vi "Thermotron 8800.vi"() -> ()   [LabVIEW 2023, in "Thermotron 8800.lvlib"]
doc: "Example vi that utilizes VISA for communication. Initializes and resets 8800 chamber controller, gets the version information, starts the chamber controller in manual mode and changes the setpoint for channel 1 process variable from zero to 10 in one degree C steps while reading back the process variable and setpoint. Finally, the chamber controller is put into stop mode, errors are handled and the example vi is closed."
uses:
  Thermotron 8800.lvlib
  Private/get set.ctl
  Private/AnalogInputChannelNumber 1-4.ctl
panel:
  in  "stop":bool
  out "Loop Count":i32
  out "PVAR1 value":string
  out "SETP1 value":string
  out "ID result":string
  out "error out":errorcluster
  in  "VISA resource name":refnum<visa-resource-name>="TCPIP::127.0.0.1::8888::SOCKET"
  in  "error in (no error)":errorcluster
  # "TCPIP::192.168.4.118::8888::SOCKET"
  # "GPIB0::1::INSTR"
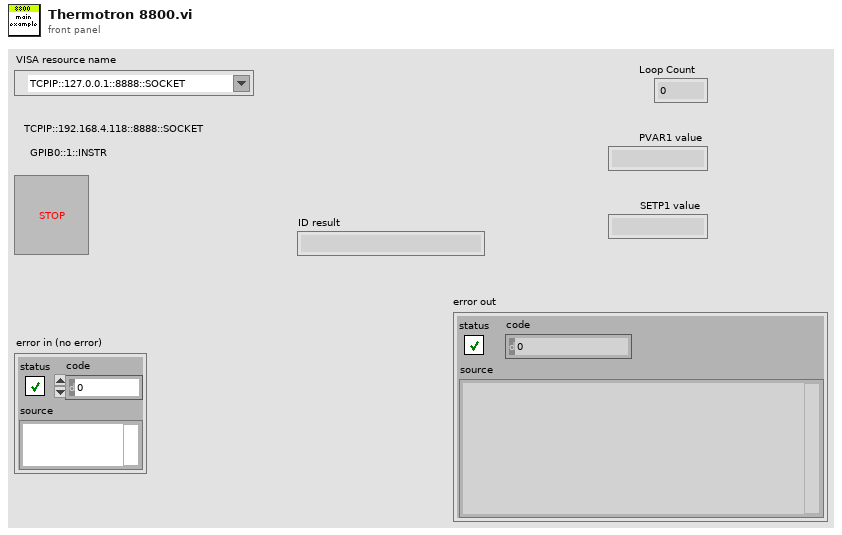
[diagram p1: front panel]
types:
  T1 = typedef "Thermotron 8800.lvlib/get set.ctl" = enum16{"get", "set"}
  T2 = typedef "Thermotron 8800.lvlib/AnalogInputChannelNumber 1-4.ctl" = u16
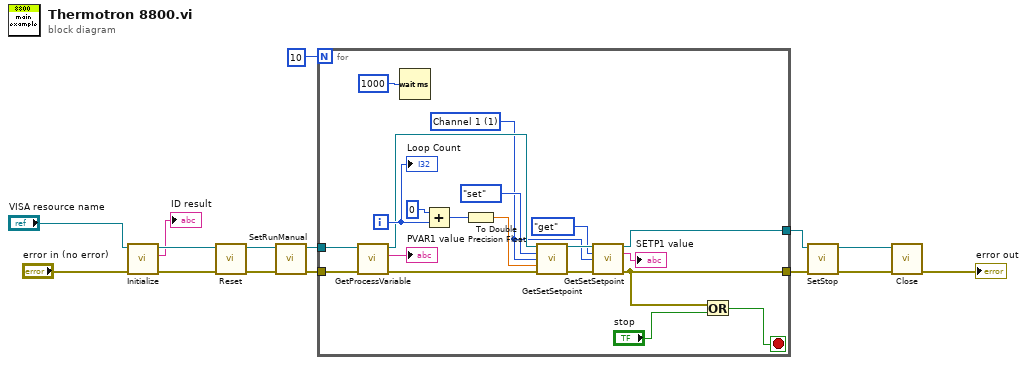
[diagram p0: block diagram]
diagram:
  n1 = call "Initialize.vi"("error in (no error)"="error in (no error)", "VISA resource name"="VISA resource name") -> ("error out"=w14:errorcluster, "ID result"=→"ID result":string, "VISA resource name out"=w15:refnum<visa-resource-name>)  [unwired: 7 in]
  n2 = call "Reset.vi"("error in (no error)"=w14, "VISA resource name"=w15) -> ("error out"=w2:errorcluster, "VISA resource name out"=w3:refnum<visa-resource-name>)  [unwired: 8 in]
  n3 = call "SetRunManual.vi"("error in"=w2, "VISA resource name"=w3) -> ("error out"=w9:errorcluster, "VISA resource name out"=w8:refnum<visa-resource-name>)  [unwired: 7 in, 1 out]
  n4 = for {
    N: 10 -> [_]
    tunnel: [w20] -> w7
    tunnel: [w16] -> w6
    tunnel: w9 -> [w32]
    tunnel: w8 -> [w31]
    i -> [w34]
    stop <- w17 stop-if-true
    w21 = T2 1 items=["Channel 1"=1, "Channel 2"=2, "Channel 3"=3, "Channel 4"=4] ("Channel Number (1-4)")
    n5 = call "GetProcessVariable.vi"("error in"=w32, "VISA resource name"=w31) -> ("error out"=w28:errorcluster, "Process Variable"=→"PVAR1 value":string, "VISA resource name out"=w29:refnum<visa-resource-name>)  [unwired: 6 in, 1 out]
    n6 = Wait (ms)(milliseconds to wait=u32 1000) -> ()  [unwired: 1 out]
    n7 = Add(x=0, y=w34) -> (x+y=w26:i32)
    n8 = To Double Precision Float(number=w26) -> (double precision float=w25:dbl)
    n9 = call "GetSetSetpoint.vi"("VISA resource name"=w29, "get/set"=get_set."set", "Channel Number (1-4)"=w21, "Setpoint"=w25, "error in"=w28) -> ("VISA resource name out"=w24:refnum<visa-resource-name>, "error out"=w23:errorcluster)  [unwired: 7 in, 2 out]
    n10 = call "GetSetSetpoint.vi"("VISA resource name"=w24, "get/set"=get_set."get", "Channel Number (1-4)"=w21, "error in"=w23) -> ("VISA resource name out"=w20:refnum<visa-resource-name>, "Setpoint string"=→"SETP1 value":string, "error out"=w16:errorcluster)  [unwired: 8 in, 1 out]
    n11 = Or(x=w16, y="stop") -> (x .or. y?=w17:bool)
    "Loop Count" <- w34
  }
  n12 = call "SetStop.vi"("error in"=w6, "VISA resource name"=w7) -> ("error out"=w4:errorcluster, "VISA resource name out"=w5:refnum<visa-resource-name>)  [unwired: 8 in]
  n13 = call "Close.vi"("error in (no error)"=w4, "VISA resource name"=w5) -> ("error out"=→"error out":errorcluster)  [unwired: 9 in]
